vi "Check Output Duplicate.vi"(0 "Input Array":u8[][](array[numeric]), 7 "New Point":u8[](array[numeric])) -> (8 "Duplicate?":bool)   [LabVIEW 2010]
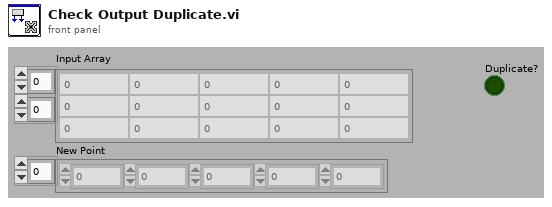
[diagram p1: front panel]
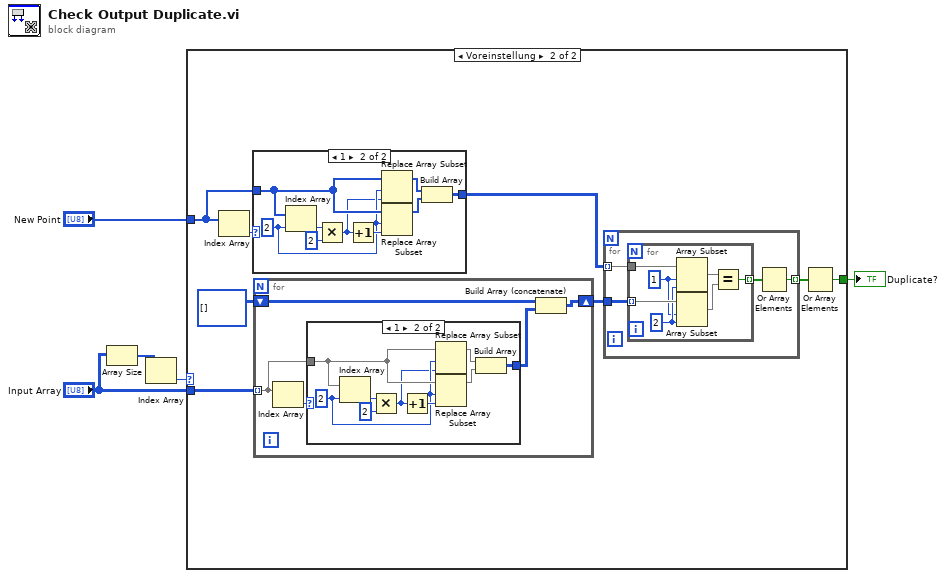
[diagram p0: block diagram]
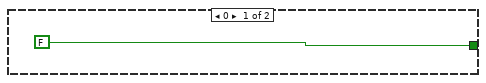
[diagram p2: hidden frame]
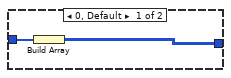
[diagram p3: hidden frame]
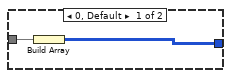
[diagram p4: hidden frame]
diagram:
  n1 = Array Size(array="Input Array") -> (size(s)=w2:i32[])
  n2 = Index Array(array=w2) -> (element=w1:i32)  [unwired: 1 in]
  n3 = case shown="Voreinstellung" w1 {
    tunnel: "New Point" -> [_ w8]
    tunnel: [FALSE w13] -> w4
    tunnel: "Input Array" -> [_ w12]
    frame 0 {
    }
    frame Default {
      n4 = Index Array(array=w8) -> (element=w9:u8)  [unwired: 1 in]
      n5 = case shown="1" w9 {
        tunnel: w8 -> [w16 w20]
        tunnel: [w15 w21] -> w7
        frame 0, Default {
          n6 = Build Array(w16) -> (w15:u8[][])
        }
        frame 1 {
          w19 = 2 ("index")
          n7 = Index Array(array=w20, index=w19) -> (element=w25:u8)
          n8 = Multiply(x=w25, y=u8 2) -> (x*y=w18:u8)
          n9 = Increment(x=w18) -> (x+1=w23:u8)
          n10 = Replace Array Subset(array=w20, new element=w18, index=w19) -> (w17:u8[])
          n11 = Replace Array Subset(array=w20, new element=w23, index=w19) -> (w22:u8[])
          n12 = Build Array(w17, w22) -> (w21:u8[][])
        }
      }
      n13 = for {
        tunnel: w12 -> [w29] mode=indexing
        shift-right: [w26] -> w10
        shift-left: u8[][] [] ("Input Array") -> [w28]
        n14 = Index Array(array=w29) -> (element=w30:u8)  [unwired: 1 in]
        n15 = case shown="1" w30 {
          tunnel: w29 -> [w32 w36]
          tunnel: [w31 w37] -> w27
          frame 0, Default {
            n16 = Build Array(w32) -> (w31:u8[][])
          }
          frame 1 {
            w35 = 2 ("index")
            n17 = Index Array(array=w36, index=w35) -> (element=w41:u8)
            n18 = Multiply(x=w41, y=u8 2) -> (x*y=w34:u8)
            n19 = Increment(x=w34) -> (x+1=w39:u8)
            n20 = Replace Array Subset(array=w36, new element=w34, index=w35) -> (w33:u8[])
            n21 = Replace Array Subset(array=w36, new element=w39, index=w35) -> (w38:u8[])
            n22 = Build Array(w33, w38) -> (w37:u8[][])
          }
        }
        n23 = Build Array (concatenate)(w28, w27) -> (w26:u8[][])
      }
      n24 = for {
        tunnel: w7 -> [w44] mode=indexing
        tunnel: w10 -> [w45]
        tunnel: [w42] -> w14 mode=indexing
        n25 = for {
          tunnel: w45 -> [w50] mode=indexing
          tunnel: w44 -> [w52]
          tunnel: [w51] -> w43 mode=indexing
          w46 = 1 ("index")
          w49 = 2 ("length")
          n26 = Array Subset(array=w52, index=w46, length=w49) -> (w48:u8[])
          n27 = Array Subset(array=w50, index=w46, length=w49) -> (w47:u8[])
          n28 = Equal?(x=w48, y=w47) -> (x = y?=w51:bool)
        }
        n29 = Or Array Elements(Boolean array=w43) -> (logical OR=w42:bool)
      }
      n30 = Or Array Elements(Boolean array=w14) -> (logical OR=w13:bool)
    }
  }
  "Duplicate?" <- w4
